vi "MVR.vi"(0 "System no.":i32=1 min=1 max=4 step=1, 2 "Axes to move":string[](array[string]), 3 "Position values":dbl[](array[numeric]) format="%.6f", 4 "No.of digits":i16=4, 5 "error in":errorcluster) -> (19 "error out":errorcluster)   [LabVIEW 2026]
doc: "Moves specified axes relative to current positions. No. of digits is the number of digits after the decimal point in the position value(s) that will be sent.\n\nC-413: Motion commands are not allowed when the wave generator is active or the analog input is used for target generation.\n\nC-867: This command works only in closed-loop operation. Motion commands like MVR are not allowed when a joystick is active on the axis.\n\nC-877: This command works only in closed-loop operation.\n\nC-880K005: VI only supported when called through PI_Multix.vi\n\nC-884: This command works only in closed-loop operation. Motion commands like MOV are not allowed when control via a Human Interface Device (HID) is active on the axis.\n\nC-891: This command works only in closed-loop operation. Motion commands are not allowed when the wave generator is active.\n\nE-517, E-518: Motion commands like MVR are not allowed when the controller is in OFFLINE mode or when the wave generator output is active. When a macro is running on the controller, MVR will be executed not until the macro is finished or stopped. See \"Control Value Generation\" and \"Control Modes\" in the controller user manual for details.\n\nE-709: Motion commands are not allowed when the wave generator is active or the analog input is used for target generation.\n\nE-710: See also NMVR.vi in Old commands.llb .\n\nE-712: Motion commands are not allowed when a wave generator is active or the analog input is used for target generation.\n\nE-725, E-727: Motion commands are not allowed when a wave generator is active or the analog input is used for target generation.\n\nE-753, E-754: Motion commands are not allowed when the wave generator is active or the analog input is used for target generation.\n\nE-755: Command not available for E-755.101.\n\nE-816: Only one axis per command allowed. It is necessary to wait a certain time before sending the next command to prevent it from being lost. \n\nE-861: This command works only in closed-loop operation. With open-loop systems, use OAD, OSM, OMA or OMR instead to command motion. Motion commands like MVR are not allowed when a joystick is active on the axis.\n\nE-871, E-873, E-874: This command works only in closed-loop operation. Motion commands like MOV are not allowed when a joystick is active on the axis.\n\nC-887, F-206, M-8X0: Only for GCS syntax version = GCS 2.0 or higher (check with CSV?.vi. If CSV?.vi is not supported, syntax version is GCS 1.0).\n\nHydra, Pollux: This command works only in closed-loop operation.\n\nMercury_GCS: This command works only in closed-loop operation. \nMotion commands like MVR are not allowed when a joystick is active on the axis."
panel:
  # "Moves stage relative to actual position."
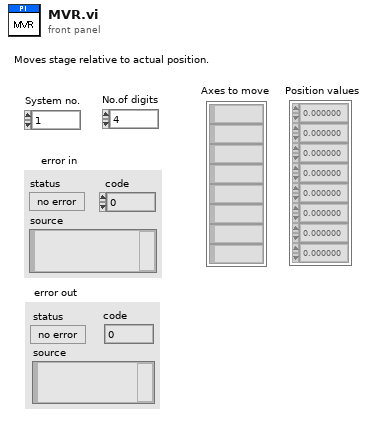
[diagram p1: front panel]
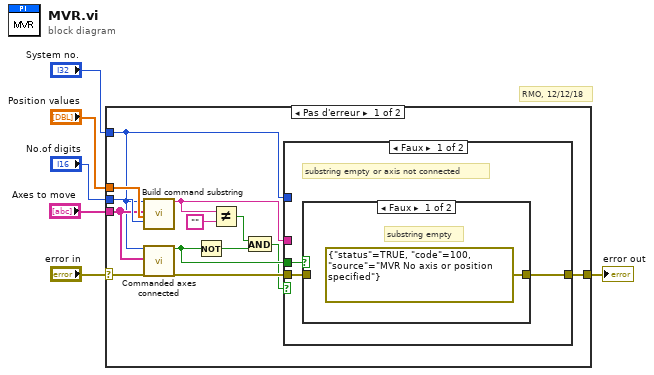
[diagram p0: block diagram]
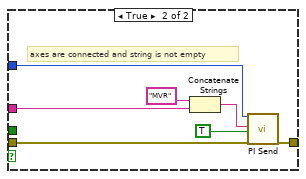
[diagram p3: hidden frame]
diagram:
  # "RMO, 12/12/18"
  n1 = case shown="Pas d'erreur" "error in" {
    selector: "error in" -> [w7 w32]
    tunnel: [w19 w32] -> w6
    tunnel: "Position values" -> [w16 _]
    tunnel: "No.of digits" -> [w15 _]
    tunnel: "System no." -> [w8 _]
    tunnel: "Axes to move" -> [w13 _]
    frame No Error {
      n2 = call "Build command substring.vi"("System no."=w8, "Affected axes"=w13, "Parameters"=w16, "No. of digits"=w15) -> ("Command substring"=w17:string)  [unwired: 3 in, 12 out]
      n3 = call "Commanded axes connected.vi"("System no."=w8, "Commanded axes"=w13, "error in"=w7) -> ("Controller error"=w11:bool, "error out"=w14:errorcluster)  [unwired: 1 in, 14 out]
      n4 = Not(x=w11) -> (.not. x?=w10:bool)
      n5 = Not Equal?(x=w17, y="") -> (x != y?=w12:bool)
      n6 = And(x=w12, y=w10) -> (x .and. y?=w9:bool)
      n7 = case shown="Faux" w9 {
        tunnel: w17 -> [_ w30]
        tunnel: [w22 w26] -> w19
        tunnel: w14 -> [w20 w27]
        tunnel: w11 -> [w21 _]
        tunnel: w8 -> [_ w25]
        frame False {
          # "substring empty or axis not connected"
          n8 = case shown="Faux" w21 {
            tunnel: [errorcluster {"status"=TRUE, "code"=100, "source"="MVR No axis or position specified"} ("error out") w24] -> w22
            tunnel: w20 -> [_ w24]
            frame False {
              # "substring empty"
            }
            frame True {
              # "commanded axis not connected"
            }
          }
        }
        frame True {
          # "axes are connected and string is not empty"
          n9 = Concatenate Strings("MVR", w30) -> (w28:string)
          n10 = call "PI Send.vi"("System no."=w25, "String to send"=w28, "Attach termination char.?"=TRUE ("Attach Linefeed?"), "error in"=w27) -> ("error out"=w26:errorcluster)  [unwired: 2 in, 13 out]
        }
      }
    }
    frame Error {
    }
  }
  "error out" <- w6
